vi "ConvertLocals.vi"(5 "PythonConverter_BD in":refnum<class "PyConvBD.lvclass">, 6 "error in":errorcluster, 9 "Diagram in":refnum<class "Diagram.lvclass">) -> (0 "error out":errorcluster, 3 "Diagram out":refnum<class "Diagram.lvclass">, 4 "PythonConverter_BD out":refnum<class "PyConvBD.lvclass">)   [LabVIEW 2014, in "Raspberry Pi Compatible Compiler for LabVIEW.lvlib" / "Diagram.lvclass"]
uses:
  Diagram.lvclass
  Python/PythonConverter_BD/PyConvBD.lvclass
  Diagram.lvclass/Diagram.ctl
  Local/Local.lvclass
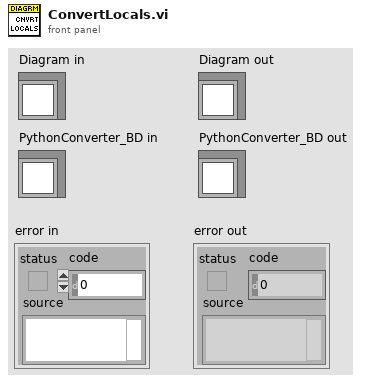
[diagram p1: front panel]
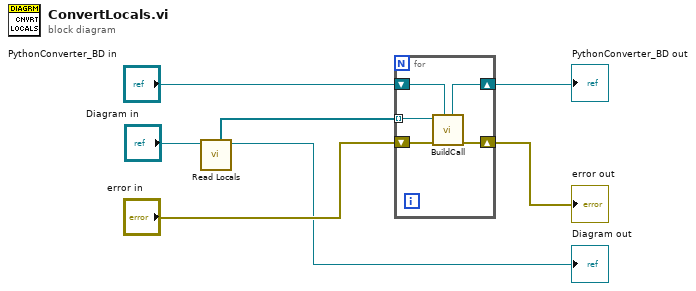
[diagram p0: block diagram]
diagram:
  n1 = call "Read Locals.vi"("Diagram in"="Diagram in") -> ("Diagram out"=→"Diagram out":refnum<class "Diagram.lvclass">, "Locals"=w2:refnum<class "Local.lvclass">[])  [unwired: 7 in]
  n2 = for {
    tunnel: w2 -> [w8] mode=indexing
    shift-right: [w11] -> w4
    shift-left: "PythonConverter_BD in" -> [w12]
    shift-right: [w9] -> w3
    shift-left: "error in" -> [w10]
    n3 = call-dynamic "BuildCall.vi"("PythonConverter_BD in"=w12, "error in"=w10, "Local in"=w8) -> ("error out"=w9:errorcluster, "PythonConverter_BD out"=w11:refnum<class "PyConvBD.lvclass">)  [unwired: 6 in, 1 out]
  }
  "error out" <- w3
  "PythonConverter_BD out" <- w4
